vi "Reset Error Log.vi"(0 "Socket Auto Connect in":refnum<class "Error Interface.lvclass">, 5 "error in (no error)":errorcluster) -> (14 "Socket Auto Connect out":refnum<class "Error Interface.lvclass">, 19 "error out":errorcluster)   [LabVIEW 2019, in "Error Interface.lvclass"]
uses:
  Error Interface.lvclass
  <vilib>/Utility/miscctls.llb/LVRowAndColumnTypeDef.ctl
  Error Interface.lvclass/Error Interface.ctl
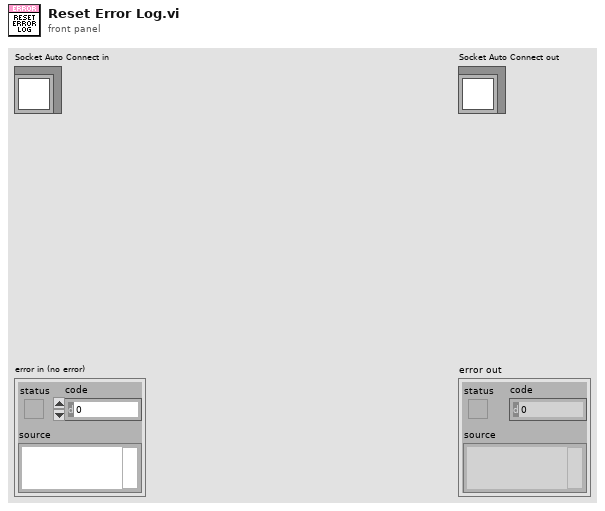
[diagram p1: front panel]
types:
  T1 = typedef "LVRowAndColumnTypeDef.ctl" = cluster{"Row":i32, "Column":i32}
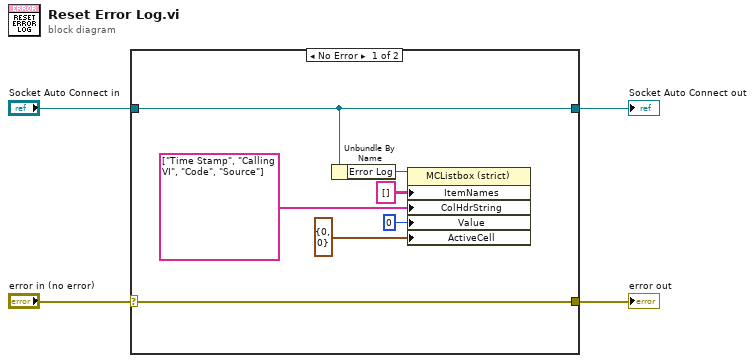
[diagram p0: block diagram]
diagram:
  n1 = case shown="No Error" "error in (no error)" {
    selector: "error in (no error)" -> [w11 w13]
    tunnel: [w11 w13] -> w3
    tunnel: [w10 w12] -> w1
    tunnel: "Socket Auto Connect in" -> [w10 w12]
    frame No Error {
      n2 = Unbundle By Name(w10) -> ("Error Log"=w9:refnum<vi>)
      n3 = property class="MCListbox (strict)"(reference=w9, "ItemNames"=string[][] [] ("Item Names"), "ColHdrString"=string[] ["Time Stamp", "Calling VI", "Code", "Source"] ("Column Header Strings[]"), "Value"=0, "ActiveCell"=T1 {"Row"=0, "Column"=0} ("Active Cell:Active Cell")) -> ()  [unwired: 1 in, 2 out]
    }
    frame Error {
    }
  }
  "error out" <- w3
  "Socket Auto Connect out" <- w1
